vi "Keithley 2450 Sweep and Acquire Measurements.vi"() -> ()   [LabVIEW 2023]
doc: "Configures a sweep and takes voltage and current readings at each point."
uses:
  Public/Data/Read (Multiple Points).vi
  Keithley 2450.lvlib
panel:
  in  "Path 2":path=path "Desktop"
  in  "Limit Level (0.1)":dbl=0.1
  in  "Delay (0) in Sec":dbl
  in  "Measurement Speed (1 PLC)":dbl=1.0 format="%.2g"
  in  "Sweep Points":T1={"Start "=1.0, "Stop "=0.0, "Number of Points (5)"=5}
  in  "Source Mode  (0: Voltage)":u16(ring) items=["Voltage", "Current"]
  in  "VISA resource name":refnum<visa-resource-name>
  out "Waveform Graph":dbl[][](graph)
  # "(c) 2021 National Instruments.  ALL RIGHTS RESERVED."
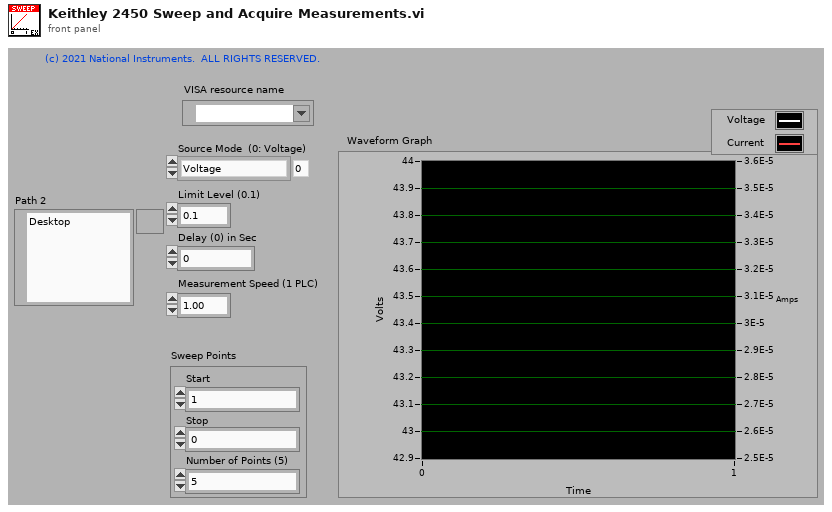
[diagram p1: front panel]
types:
  T1 = cluster{"Start ":dbl, "Stop ":dbl, "Number of Points (5)":u32}
  T2 = enum16{"open", "replace", "create", "open or create", "replace or create", "replace or create with confirmation"}
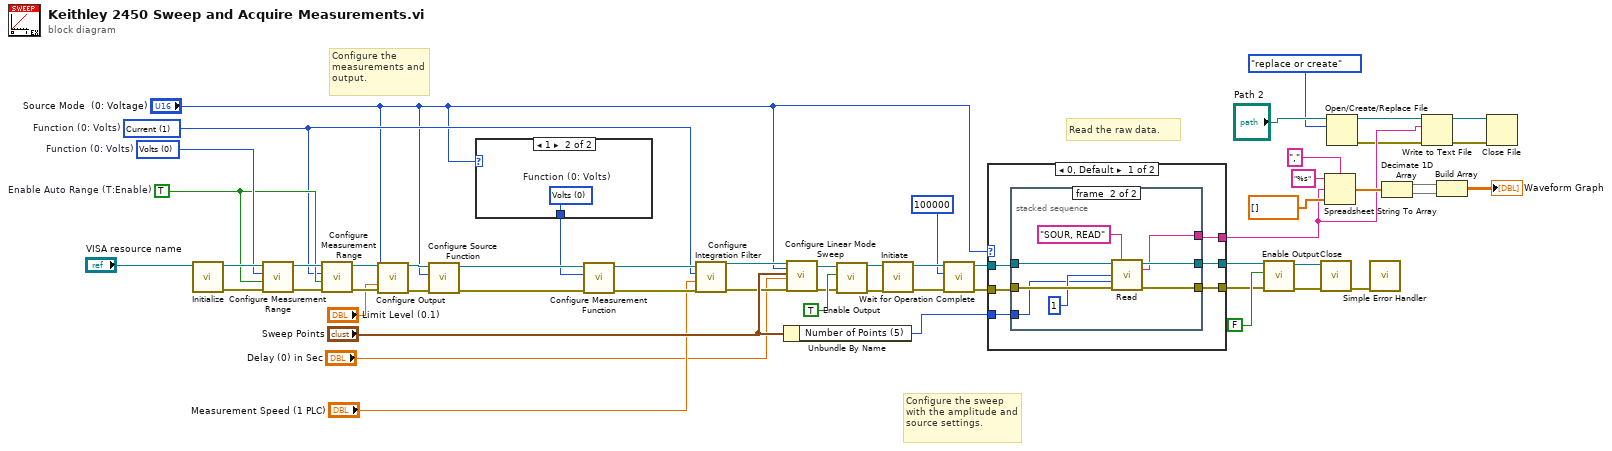
[diagram p0: block diagram]
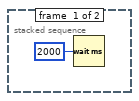
[diagram p2: hidden frame]
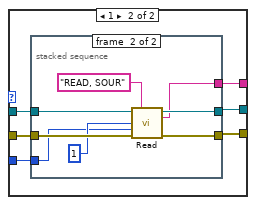
[diagram p3: hidden frame]
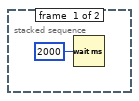
[diagram p4: hidden frame]
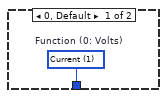
[diagram p5: hidden frame]
diagram:
  w45 = TRUE  # Enable Auto Range (T:Enable)
  w18 = u16 1 items=["Volts", "Current", "Resistance"]  # Function (0: Volts)
  w46 = u16 0 items=["Volts", "Current", "Resistance"]  # Function (0: Volts)
  # "Read the raw data."
  # "Configure the sweep with the amplitude and source settings."
  # "Configure the measurements and output."
  n1 = call "Initialize.vi"("VISA resource name"="VISA resource name") -> ("error out"=w54:errorcluster, "VISA resource name out"=w55:refnum<visa-resource-name>)  [unwired: 9 in]
  n2 = call "Configure Measurement Range.vi"("error in (no error)"=w54, "Enable Auto Range (T:Enable)"=w45, "Function (0: Volts)"=w46, "VISA resource name"=w55) -> ("error out"=w53:errorcluster, "VISA resource name out"=w52:refnum<visa-resource-name>)  [unwired: 6 in]
  n3 = call "Configure Measurement Range.vi"("error in (no error)"=w53, "Enable Auto Range (T:Enable)"=w45, "Function (0: Volts)"=w18, "VISA resource name"=w52) -> ("error out"=w42:errorcluster, "VISA resource name out"=w43:refnum<visa-resource-name>)  [unwired: 6 in]
  n4 = call "Configure Output.vi"("VISA resource name"=w43, "Source Mode  (0: Voltage)"="Source Mode  (0: Voltage)", "Source Limit Level (0.1)"="Limit Level (0.1)", "error in (no error)"=w42) -> ("VISA resource name out"=w40:refnum<visa-resource-name>, "error out"=w41:errorcluster)  [unwired: 10 in]
  n5 = call "Configure Source Function.vi"("error in (no error)"=w41, "Function (0: Volts)"="Source Mode  (0: Voltage)", "VISA resource name"=w40) -> ("error out"=w21:errorcluster, "VISA resource name out"=w22:refnum<visa-resource-name>)  [unwired: 7 in]
  n6 = case shown="1" "Source Mode  (0: Voltage)" {
    tunnel: [w56 w57] -> w17
    frame 0, Default {
      w56 = u16 1 items=["Volts", "Current", "Resistance"]  # Function (0: Volts)
    }
    frame 1 {
      w57 = u16 0 items=["Volts", "Current", "Resistance"]  # Function (0: Volts)
    }
  }
  n7 = call "Configure Measurement Function.vi"("error in (no error)"=w21, "Function (0: Volts)"=w17, "VISA resource name"=w22) -> ("error out"=w20:errorcluster, "VISA resource name out"=w19:refnum<visa-resource-name>)  [unwired: 7 in]
  n8 = call "Configure Integration Filter.vi"("error in (no error)"=w20, "Measurement Speed (1 PLC)"="Measurement Speed (1 PLC)", "Function (0: Volts)"=w18, "VISA resource name"=w19) -> ("error out"=w25:errorcluster, "VISA resource name out"=w24:refnum<visa-resource-name>)  [unwired: 6 in]
  n9 = Unbundle By Name("Sweep Points") -> ("Number of Points (5)"=w11:u32)
  n10 = call "Configure Linear Mode Sweep.vi"("VISA resource name"=w24, "Source Mode  (0: Voltage)"="Source Mode  (0: Voltage)", "Sweep Points"="Sweep Points", "Delay (0)"="Delay (0) in Sec", "error in (no error)"=w25) -> ("VISA resource name out"=w39:refnum<visa-resource-name>, "error out"=w38:errorcluster)  [unwired: 13 in]
  n11 = call "Enable Output.vi"("error in (no error)"=w38, "Enable Output (T: Enable)"=TRUE, "VISA resource name"=w39) -> ("error out"=w36:errorcluster, "VISA resource name out"=w37:refnum<visa-resource-name>)  [unwired: 7 in]
  n12 = call "Initiate.vi"("error in (no error)"=w36, "VISA resource name"=w37) -> ("error out"=w26:errorcluster, "VISA resource name out"=w27:refnum<visa-resource-name>)  [unwired: 8 in]
  n13 = call "Wait for Operation Complete.vi"("error in (no error)"=w26, "Timeout (10000 ms)"=100000, "VISA resource name"=w27) -> ("error out"=w14:errorcluster, "VISA resource name out"=w15:refnum<visa-resource-name>)  [unwired: 7 in]
  n14 = case shown="0, Default" "Source Mode  (0: Voltage)" {
    tunnel: w15 -> [w63 w78]
    tunnel: w14 -> [w62 w77]
    tunnel: [w61 w75] -> w13
    tunnel: [w60 w74] -> w12
    tunnel: w11 -> [w59 w76]
    tunnel: [w58 w73] -> w7
    frame 0, Default {
      n15 = stacked-sequence {
        tunnel: [_ w72] -> w61
        tunnel: [_ w71] -> w60
        tunnel: w63 -> [_ w69]
        tunnel: w62 -> [_ w68]
        tunnel: [_ w67] -> w58
        tunnel: w59 -> [_ w65]
        frame #0 {
          n16 = Wait (ms)(milliseconds to wait=u32 2000) -> ()  [unwired: 1 out]
        }
        frame #1 {
          n17 = call-poly "Read.vi"("VISA resource name"=w69, "Buffer Elements"="SOUR, READ", "Start Index (1)"=1, "End Index (1)"=w65, "error in (no error)"=w68) -> ("VISA resource name out"=w72:refnum<visa-resource-name>, "Data out"=w67:string, "error out"=w71:errorcluster)  [unwired: 8 in]
        }
      }
    }
    frame 1 {
      n18 = stacked-sequence {
        tunnel: [_ w87] -> w75
        tunnel: [_ w86] -> w74
        tunnel: w78 -> [_ w84]
        tunnel: w77 -> [_ w83]
        tunnel: [_ w82] -> w73
        tunnel: w76 -> [_ w80]
        frame #0 {
          n19 = Wait (ms)(milliseconds to wait=u32 2000) -> ()  [unwired: 1 out]
        }
        frame #1 {
          n20 = call-poly "Read.vi"("VISA resource name"=w84, "Buffer Elements"="READ, SOUR", "Start Index (1)"=1, "End Index (1)"=w80, "error in (no error)"=w83) -> ("VISA resource name out"=w87:refnum<visa-resource-name>, "Data out"=w82:string, "error out"=w86:errorcluster)  [unwired: 8 in]
        }
      }
    }
  }
  n21 = call "Enable Output.vi"("error in (no error)"=w12, "Enable Output (T: Enable)"=FALSE, "VISA resource name"=w13) -> ("error out"=w48:errorcluster, "VISA resource name out"=w49:refnum<visa-resource-name>)  [unwired: 7 in]
  n22 = call "Close.vi"("error in (no error)"=w48, "VISA resource name"=w49) -> ("error out"=w50:errorcluster)  [unwired: 9 in]
  n23 = Spreadsheet String To Array(delimiter (Tab)=",", format string="%s", spreadsheet string=w7, array type (2D Dbl)=dbl[] []) -> (array=w31:dbl[])
  n24 = Open/Create/Replace File(file path (use dialog)="Path 2", operation (0:open)=T2."replace or create") -> (refnum out=w2:refnum<file>, error out=w6:errorcluster)  [unwired: 4 in, 1 out]
  n25 = call <vilib>:"Simple Error Handler.vi"("error in (no error)"=w50) -> ()  [unwired: 4 in, 5 out]
  n26 = Decimate 1D Array(w31) -> (w30:dbl[], w29:dbl[])
  n27 = Write to Text File(file (use dialog)=w2, text=w7, error in=w6) -> (refnum out=w4:refnum<file>, error out=w5:errorcluster)  [unwired: 1 in, 1 out]
  n28 = Build Array(w30, w29) -> (→"Waveform Graph":dbl[][])
  n29 = Close File(refnum=w4, error in=w5) -> ()  [unwired: 2 out]
